vi "MainPage.vi"(7 "LabVIEW Web Service Request":refnum<class "Web Request.lvclass">) -> ()   [LabVIEW 2018]
uses:
  <vilib>/wsapi/Web Request.lvclass
  Type def mainpage.ctl
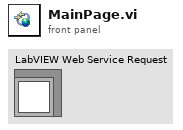
[diagram p1: front panel]
types:
  T1 = typedef "Type def mainpage.ctl" = cluster{"Valve Status":bool, "Pressure Status":bool, "Hutch Status":bool, "Flow Rate Status":bool, "Temperature Status ":bool, "BL1.1W Shutter":bool, "Beam Current":sgl, "Injection Status":i16, "XAS Status":bool, "Auto Fill Status":bool, "LN2 Level":dbl, "XAS Mode":u8}
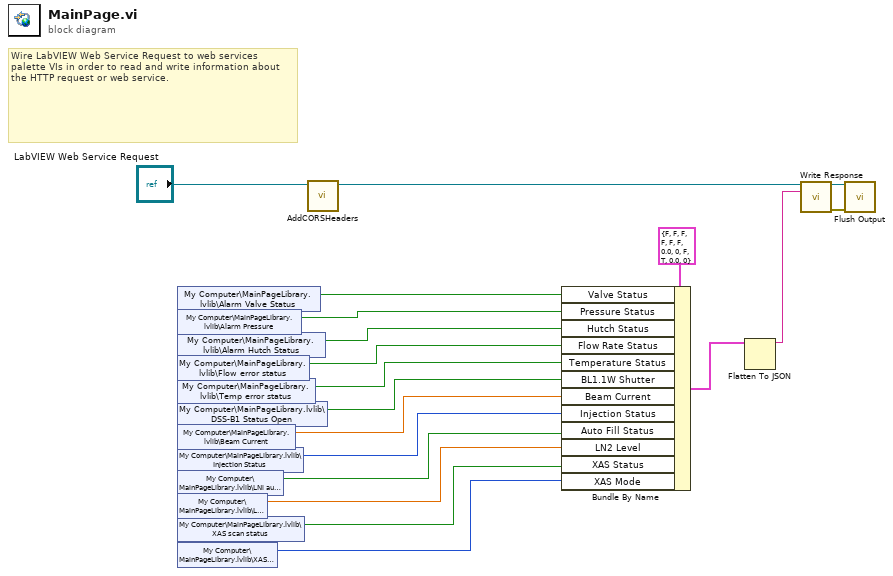
[diagram p0: block diagram]
diagram:
  # "Wire LabVIEW Web Service Request to web services palette VIs in order to read and write information about the HTTP request or web service."
  n1 = shared-variable "My Computer\\MainPageLibrary.lvlib\\Alarm Valve Status"() -> (w4:bool)  [unwired: 1 in, 1 out]
  n2 = shared-variable "My Computer\\MainPageLibrary.lvlib\\Alarm Pressure"() -> (w10:bool)  [unwired: 1 in, 1 out]
  n3 = shared-variable "My Computer\\MainPageLibrary.lvlib\\Alarm Hutch Status"() -> (w3:bool)  [unwired: 1 in, 1 out]
  n4 = shared-variable "My Computer\\MainPageLibrary.lvlib\\Flow error status"() -> (w9:bool)  [unwired: 1 in, 1 out]
  n5 = shared-variable "My Computer\\MainPageLibrary.lvlib\\Temp error status"() -> (w8:bool)  [unwired: 1 in, 1 out]
  n6 = shared-variable "My Computer\\MainPageLibrary.lvlib\\DSS-B1 Status Open"() -> (w2:bool)  [unwired: 1 in, 1 out]
  n7 = shared-variable "My Computer\\MainPageLibrary.lvlib\\Beam Current"() -> (w14:sgl)  [unwired: 1 in, 1 out]
  n8 = shared-variable "My Computer\\MainPageLibrary.lvlib\\Injection Status"() -> (w13:i16)  [unwired: 1 in, 1 out]
  n9 = shared-variable "My Computer\\MainPageLibrary.lvlib\\LNi auto fill"() -> (w12:bool)  [unwired: 1 in, 1 out]
  n10 = shared-variable "My Computer\\MainPageLibrary.lvlib\\LNi level"() -> (w11:dbl)  [unwired: 1 in, 1 out]
  n11 = shared-variable "My Computer\\MainPageLibrary.lvlib\\XAS scan status"() -> (w7:bool)  [unwired: 1 in, 1 out]
  n12 = shared-variable "My Computer\\MainPageLibrary.lvlib\\XAS Mode"() -> (w1:u8)  [unwired: 1 in, 1 out]
  n13 = call "AddCORSHeaders.vi"("Web Request in"="LabVIEW Web Service Request") -> ("Web Request out"=w6:refnum<class "Web Request.lvclass">)  [unwired: 10 in]
  n14 = Bundle By Name(cluster=T1 {"Valve Status"=FALSE, "Pressure Status"=FALSE, "Hutch Status"=FALSE, "Flow Rate Status"=FALSE, "Temperature Status "=FALSE, "BL1.1W Shutter"=FALSE, "Beam Current"=0.0, "Injection Status"=0, "XAS Status"=FALSE, "Auto Fill Status"=TRUE, "LN2 Level"=0.0, "XAS Mode"=0} ("Cluster"), "Valve Status"=w4, "Pressure Status"=w10, "Hutch Status"=w3, "Flow Rate Status"=w9, "Temperature Status"=w8, "BL1.1W Shutter"=w2, "Beam Current"=w14, "Injection Status"=w13, "Auto Fill Status"=w12, "LN2 Level"=w11, "XAS Status"=w7, "XAS Mode"=w1) -> (w15:T1)
  n15 = Flatten To JSON(anything=w15) -> (JSON string=w16:string)  [unwired: 2 in, 1 out]
  n16 = call <vilib>:"Write Response.vi"("LabVIEW Web Service Request"=w6, "response string"=w16) -> ("LabVIEW Web Service Request out"=w19:refnum<class "Web Request.lvclass">, "error out"=w18:errorcluster)  [unwired: 12 in]
  n17 = call <vilib>:"Flush Output.vi"("LabVIEW Web Service Request"=w19, "error in (no error)"=w18) -> ()  [unwired: 12 in, 2 out]
